vi "PH_TKTDS-30xx.panel.vi"(0 "object ref":refnum<vi>, 5 "error in (no error)":errorcluster) -> (19 "error out":errorcluster)   [LabVIEW 2014, in "PH_TKTDS-30xx.lvlib"]
doc: "This a GUI.\n\nLicense Agreement for this software:\n\nCopyright (C)\nGesellschaft für Schwerionenforschung, GSI\nPlanckstr. 1\n64291 Darmstadt\nGermany\n\nContact: D.Beck@gsi.de \n\nThis program is free software; you can redistribute it and/or modify it under the terms of the GNU General Public License as published by the Free Software Foundation; either version 2 of the license, or (at your option) any later version.\n\nThis program is distributed in the hope that it will be useful, but WITHOUT ANYW ARRANTY; without even the implied warranty of MERCHANTABILITY or FITNESS FOR A PARTICULAR PURPOSE. See the GNU General License for more details (http://www.gnu.org).\n\nGesellschaft für Schwerionenforschung, GSI\nPlanckstr. 1, 64291 Darmstadt, Germany\nFor all questions and ideas contact: M.Richter@gsi.de, H.Brand@gsi.de or D.Beck@gsi.de.\nLast update: 18-DEC-2002"
uses:
  PH_TKTDS-30xx.lvlib
  PH_TKTDS-30xx.Channel Config.ctl
  PH_TKTDS-30xx.Waveform Limits.ctl
  PH_TKTDS-30xx.Acquisition Config.ctl
  PH_TKTDS-30xx.Trigger Config.ctl
  PH_TKTDS-30xx.GUI Refs.ctl
  CS_Core/CSObj/CSObj.lvlib
  PH_Basics/PH_Common/PH_Common.lvlib
  CS_Core/CSSystem/CSSystemLib/CSSystemLib.lvlib
  PH_Basics/PH_Class/PH_Class.lvlib
panel:
  out "VISA Resource":string
  out "State":u32(colorbox)
  in  "Tab Control":T1(tab)
  out "Graph":waveform(dbl)[](graph)
  in  "Trigger":T2={"Source"="CH1", "Slope"=0, "Level [V]"=0.0} {"Level [V]" format="%#_6p"}
  in  "Acquisition":T3={"Time base"=2e-07, "Record Length"=10000, "Start Time"=0.0, "Type"=0, "Continuous"=FALSE} {"Start Time" format="%#_12p"; "Record Length" items=["500"=500, "10000"=10000]; "Time base" items=["2ns"=2e-09, "4ns"=4e-09, "10ns"=1e-08, "20ns"=2e-08, "40ns"=4e-08, "100ns"=1e-07, "200ns"=2e-07, "400ns"=4e-07, "1µs"=1e-06, "2µs"=2e-06, "4µs"=4e-06, "10µs"=1e-05, "20µs"=2e-05, "40µs"=4e-05, "100µs"=0.0001, "200µs"=0.0002, "400µs"=0.0004, "1ms"=0.001, "2ms"=0.002, "10ms"=0.01, "20ms"=0.02, "40ms"=0.04, "100ms"=0.1, "200ms"=0.2, "400ms"=0.4, "1s"=1.0, "2s"=2.0, "4s"=4.0, "10s"=10.0]}
  in  "Signal 2":T4={"Channel Name"="CH1", "Input Impedance"="MEG", "Max Input Frequency"="TWENTY", "Vertical Coupling"=1, "Channel Enabled"=TRUE, "Probe Attenuation"=1.0, "Vertical Range"=100.0, "Vertical Offset"=0.0, "Waveform Limits"={"Start"=1, "End"=10000}} {"Vertical Offset" format="%#_6p"; "Vertical Range" items=["1mV"=0.001, "2mV"=0.002, "5mV"=0.005, "10mV"=0.01, "20mV"=0.02, "50mV"=0.05, "100mV"=0.1, "200mV"=0.2, "500mV"=0.5, "1V"=1.0]; "Probe Attenuation" format="%#.2f"}
  in  "Signal 1":T4={"Channel Name"="CH1", "Input Impedance"="MEG", "Max Input Frequency"="TWENTY", "Vertical Coupling"=1, "Channel Enabled"=TRUE, "Probe Attenuation"=1.0, "Vertical Range"=100.0, "Vertical Offset"=0.0, "Waveform Limits"={"Start"=1, "End"=10000}} {"Vertical Offset" format="%#_6p"; "Vertical Range" items=["1mV"=0.001, "2mV"=0.002, "5mV"=0.005, "10mV"=0.01, "20mV"=0.02, "50mV"=0.05, "100mV"=0.1, "200mV"=0.2, "500mV"=0.5, "1V"=1.0]; "Probe Attenuation" format="%#.2f"}
  in  "Display Intensity":u8=1 min=1 max=100 step=1
  in  "Channel to be positioned":string(combo)="CH1"
  in  "Position":dbl
  out "PSDB Status":u32(colorbox)=6618880 caption="PSDB"
  in  "Delete":bool
  in  "Exit":bool
  # "PCS"
  # "3.40"
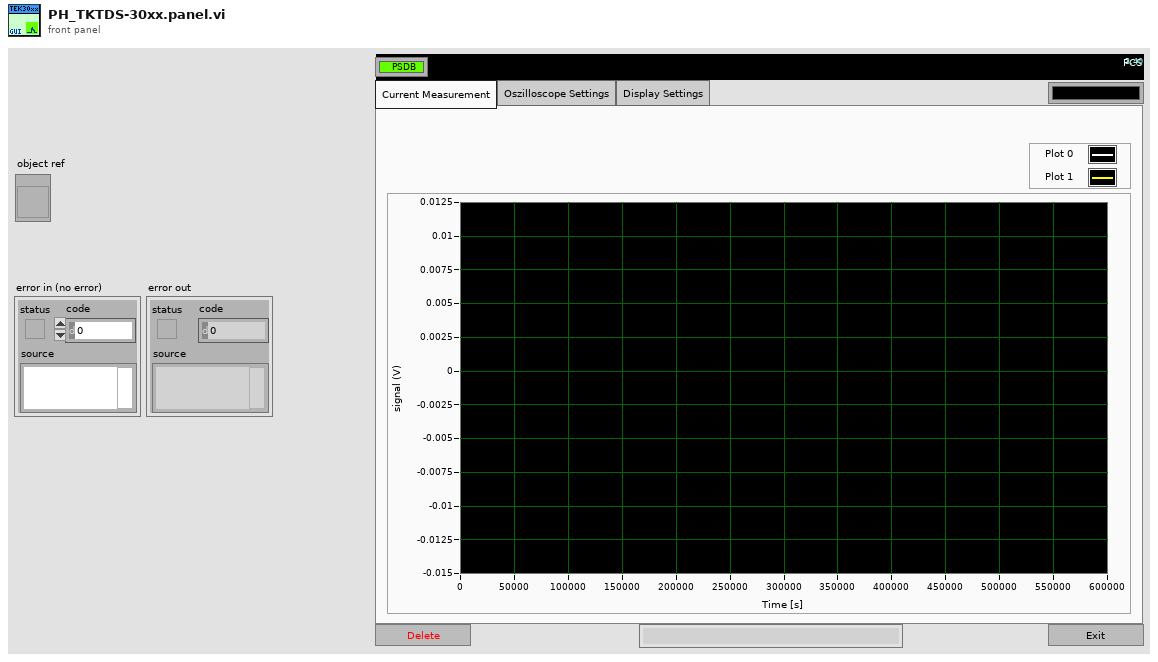
[diagram p1: front panel]
types:
  T1 = enum32{"Current Measurement", "Oszilloscope Settings", "Display Settings"}
  T2 = typedef "PH_TKTDS-30xx.lvlib/PH_TKTDS-30xx.Trigger Config.ctl" = cluster{"Source":string, "Slope":i32, "Level [V]":dbl}
  T3 = typedef "PH_TKTDS-30xx.lvlib/PH_TKTDS-30xx.Acquisition Config.ctl" = cluster{"Time base":dbl, "Record Length":u16, "Start Time":dbl, "Type":i32, "Continuous":bool}
  T4 = typedef "PH_TKTDS-30xx.lvlib/PH_TKTDS-30xx.Channel Config.ctl" = cluster{"Channel Name":string, "Input Impedance":string, "Max Input Frequency":string, "Vertical Coupling":i32, "Channel Enabled":bool, "Probe Attenuation":dbl, "Vertical Range":dbl, "Vertical Offset":dbl, "Waveform Limits":T5}
  T5 = typedef "PH_TKTDS-30xx.lvlib/PH_TKTDS-30xx.Waveform Limits.ctl" = cluster{"Start":i32, "End":i32}
  T6 = typedef "PH_TKTDS-30xx.lvlib/PH_TKTDS-30xx.GUI Refs.ctl" = cluster{"Trigger":refnum<vi>, "Acquisition":refnum<vi>, "State":refnum<vi>, "Delete":refnum<vi>, "Channel to be positioned":refnum<vi>, "Postion":refnum<vi>, "Display Intensity":refnum<vi>, "VISA Resource":refnum<vi>, "Channels":refnum<vi>[], "Graphs":refnum<vi>[]}
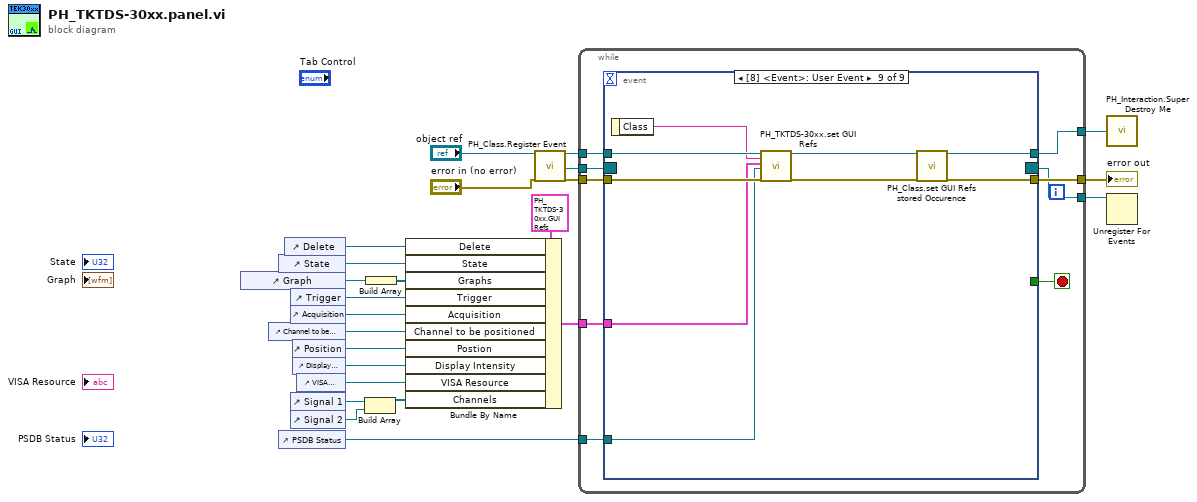
[diagram p0: block diagram]
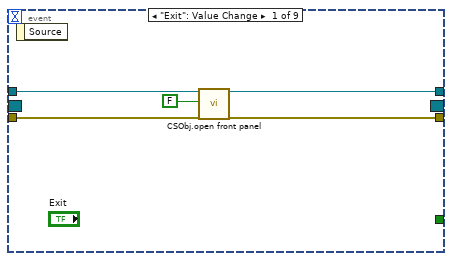
[diagram p2: hidden frame]
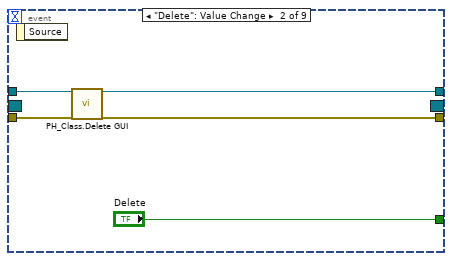
[diagram p3: hidden frame]
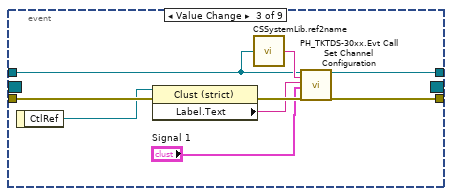
[diagram p4: hidden frame]
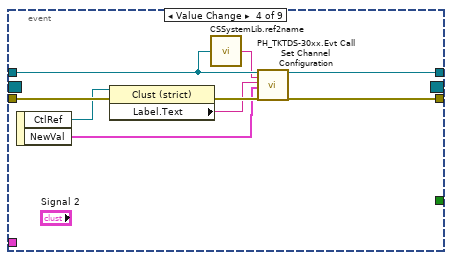
[diagram p5: hidden frame]
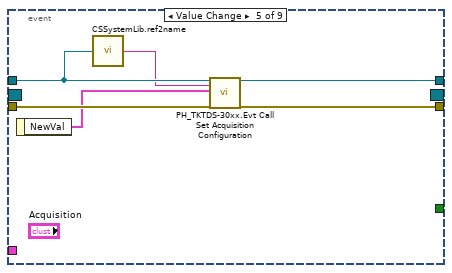
[diagram p6: hidden frame]
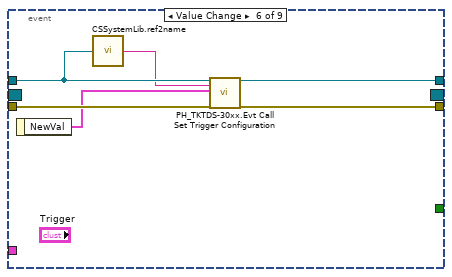
[diagram p7: hidden frame]
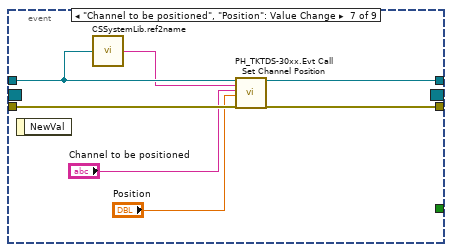
[diagram p8: hidden frame]
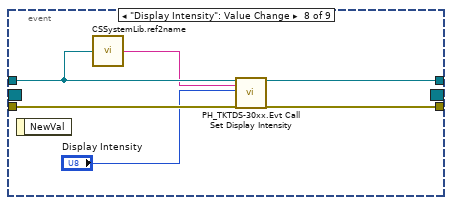
[diagram p9: hidden frame]
diagram:
  n1 = control-ref of="Graph"() -> (w20:refnum<vi>)
  n2 = control-ref of="Channel to be positioned"() -> (w16:refnum<vi>)
  n3 = control-ref of="State"() -> (w21:refnum<vi>)
  n4 = control-ref of="PSDB Status"() -> (w2:refnum<vi>)
  n5 = control-ref of="Delete"() -> (w22:refnum<vi>)
  n6 = control-ref of="Trigger"() -> (w18:refnum<vi>)
  n7 = control-ref of="Acquisition"() -> (w19:refnum<vi>)
  n8 = control-ref of="Signal 1"() -> (w1:refnum<vi>)
  n9 = control-ref of="Signal 2"() -> (w17:refnum<vi>)
  n10 = control-ref of="Position"() -> (w15:refnum<vi>)
  n11 = control-ref of="Display Intensity"() -> (w14:refnum<vi>)
  n12 = control-ref of="VISA Resource"() -> (w13:refnum<vi>)
  n13 = Build Array(w1, w17) -> (w8:refnum<vi>[])
  n14 = Build Array(w20) -> (w4:refnum<vi>[])
  n15 = Bundle By Name(cluster=T6 {"Trigger"=refnum, "Acquisition"=refnum, "State"=refnum, "Delete"=refnum, "Channel to be positioned"=refnum, "Postion"=refnum, "Display Intensity"=refnum, "VISA Resource"=refnum, "Channels"=[], "Graphs"=[]} ("GUI Refs"), "Delete"=w22, "State"=w21, "Graphs"=w4, "Trigger"=w18, "Acquisition"=w19, "Channel to be positioned"=w16, "Postion"=w15, "Display Intensity"=w14, "VISA Resource"=w13, "Channels"=w8) -> (w5:T6)
  n16 = call "PH_Class.Register Event.vi"("i ref in"="object ref", "error in (no error)"="error in (no error)") -> ("i ref out"=w12:refnum<vi>, "Event Registration Refnum"=w10:refnum<event-registration>, "error out"=w11:errorcluster)  [unwired: 15 in]
  n17 = while {
    tunnel: w12 -> [w30]
    tunnel: [w29] -> w24
    tunnel: w11 -> [w32]
    tunnel: [w31] -> w23
    tunnel: w10 -> [w28]
    tunnel: [w27] -> w9
    tunnel: w5 -> [w26]
    tunnel: w2 -> [w25]
    stop <- w33 stop-if-true
    n18 = event shown="[8] <Event>: User Event" {
      selector: w28 -> [_ _ _ _ _ _ _ _ _]
      dyn-events: [_ _ _ _ _ _ _ _ _] -> w27
      timeout: _ -> [_ _ _ _ _ _ _ _ _]
      tunnel: [_ "Delete" _ _ _ _ _ _ _] -> w33
      tunnel: w30 -> [w35 w41 w47 w58 w64 w70 w77 w83 w95]
      tunnel: w32 -> [w38 w42 w49 w61 w67 w73 w80 w86 w93]
      tunnel: [w37 w39 w48 w60 w66 w72 w79 w85 w90] -> w31
      tunnel: [w34 w40 w46 w59 w65 w71 w78 w84 w91] -> w29
      tunnel: w26 -> [_ _ _ _ _ _ _ _ w88]
      tunnel: w25 -> [_ _ _ _ _ _ _ _ w87]
      event "Exit": Value Change {
        n19 = event-data() -> ()  [unwired: 1 in, 1 out]
        n20 = call "CSObj.open front panel.vi"("i ref in"=w35, "frontPanelOpen"=FALSE ("front panel open"), "error in (no error)"=w38) -> ("i ref out"=w34:refnum<vi>, "error out"=w37:errorcluster)  [unwired: 15 in]
      }
      event "Delete": Value Change {
        n21 = event-data() -> ()  [unwired: 1 in, 1 out]
        n22 = call "PH_Class.Delete GUI.vi"("VI in"=w41, "error in (no error)"=w42) -> ("VI out"=w40:refnum<vi>, "error out"=w39:errorcluster)  [unwired: 16 in]
      }
      event Value Change {
        n23 = event-data() -> ("CtlRef"=w44:refnum<vi>)  [unwired: 1 in]
        n24 = property class="Clust (strict)"(reference=w44, error in=w49) -> (error out=w51:errorcluster, "Label.Text"=w50:string)  [unwired: 1 out]
        n25 = call "CSSystemLib.ref2name.vi"("obj refnum"=w47) -> ("name"=w52:string)
        n26 = call "PH_TKTDS-30xx.Evt Call Set Channel Configuration.vi"("i ref in"=w47, "Instance"=w52, "GUI Element Name"=w50, "Channel Configuration"="Signal 1", "error in (no error)"=w51) -> ("i ref out"=w46:refnum<vi>, "error out"=w48:errorcluster)  [unwired: 13 in]
      }
      event Value Change {
        n27 = event-data() -> ("CtlRef"=w55:refnum<vi>, "NewVal"=w53:T4)  [unwired: 1 in]
        n28 = property class="Clust (strict)"(reference=w55, error in=w61) -> (error out=w56:errorcluster, "Label.Text"=w54:string)  [unwired: 1 out]
        n29 = call "CSSystemLib.ref2name.vi"("obj refnum"=w58) -> ("name"=w57:string)
        n30 = call "PH_TKTDS-30xx.Evt Call Set Channel Configuration.vi"("i ref in"=w58, "Instance"=w57, "GUI Element Name"=w54, "Channel Configuration"=w53, "error in (no error)"=w56) -> ("i ref out"=w59:refnum<vi>, "error out"=w60:errorcluster)  [unwired: 13 in]
      }
      event Value Change {
        n31 = event-data() -> ("NewVal"=w62:T3)  [unwired: 1 in]
        n32 = call "CSSystemLib.ref2name.vi"("obj refnum"=w64) -> ("name"=w63:string)
        n33 = call "PH_TKTDS-30xx.Evt Call Set Acquisition Configuration.vi"("i ref in"=w64, "Instance"=w63, "Acquisition Configuration"=w62, "error in (no error)"=w67) -> ("i ref out"=w65:refnum<vi>, "error out"=w66:errorcluster)  [unwired: 14 in]
      }
      event Value Change {
        n34 = event-data() -> ("NewVal"=w68:T2)  [unwired: 1 in]
        n35 = call "CSSystemLib.ref2name.vi"("obj refnum"=w70) -> ("name"=w69:string)
        n36 = call "PH_TKTDS-30xx.Evt Call Set Trigger Configuration.vi"("i ref in"=w70, "Instance"=w69, "Trigger Configuration"=w68, "error in (no error)"=w73) -> ("i ref out"=w71:refnum<vi>, "error out"=w72:errorcluster)  [unwired: 14 in]
      }
      event "Channel to be positioned", "Position": Value Change {
        n37 = event-data() -> ()  [unwired: 1 in, 1 out]
        n38 = call "CSSystemLib.ref2name.vi"("obj refnum"=w77) -> ("name"=w76:string)
        n39 = call "PH_TKTDS-30xx.Evt Call Set Channel Position.vi"("i ref in"=w77, "Instance"=w76, "Channel to be positioned"="Channel to be positioned", "Position"="Position", "error in (no error)"=w80) -> ("i ref out"=w78:refnum<vi>, "error out"=w79:errorcluster)  [unwired: 13 in]
      }
      event "Display Intensity": Value Change {
        n40 = event-data() -> ()  [unwired: 1 in, 1 out]
        n41 = call "CSSystemLib.ref2name.vi"("obj refnum"=w83) -> ("name"=w82:string)
        n42 = call "PH_TKTDS-30xx.Evt Call Set Display Intensity.vi"("i ref in"=w83, "Instance"=w82, "Display Intensity"="Display Intensity", "error in (no error)"=w86) -> ("i ref out"=w84:refnum<vi>, "error out"=w85:errorcluster)  [unwired: 14 in]
      }
      event User Event {
        n43 = event-data() -> ("Class"=w89:string)  [unwired: 1 in]
        n44 = call "PH_TKTDS-30xx.set GUI Refs.vi"("i ref in"=w95, "Class"=w89, "GUI Refs"=w88, "Ref PSDB Status"=w87, "error in (no error)"=w93) -> ("i ref out"=w94:refnum<vi>, "error out"=w92:errorcluster)  [unwired: 13 in]
        n45 = call "PH_Class.set GUI Refs stored Occurence.vi"("i ref in"=w94, "error in (no error)"=w92) -> ("i ref out"=w91:refnum<vi>, "error out"=w90:errorcluster)  [unwired: 16 in]
      }
    }
  }
  "error out" <- w23
  n46 = call "PH_Interaction.Super Destroy Me.vi"("i ref out"=w24) -> ()
  n47 = Unregister For Events(event registration refnum=w9) -> ()  [unwired: 1 in, 1 out]
